vi "Do Something.vi"(8 "error in (no error)":errorcluster, 10 "Bytes to Read":i32, 11 "Inst.Xeryon-Rotator in":refnum<class "Inst.Xeryon-Rotator.lvclass">) -> (0 "error out":errorcluster, 3 "Inst.Xeryon-Rotator out":refnum<class "Inst.Xeryon-Rotator.lvclass">)   [LabVIEW 2019, in "Inst.Xeryon-Rotator.lvclass"]
uses:
  Inst.Xeryon-Rotator.lvclass
  Typedefs/Inst.Xeryon-Rotator.Commands--Enum.ctl
  <userlib>/LevyLab/Instrument Framework/Instrument/Instrument.lvclass
  C:/Program Files (x86)/National Instruments/LabVIEW 2019/user.lib/LevyLab/Instrument Framework/Instrument Types/Cryostat/Instrument.Cryostat.lvclass
  C:/Program Files (x86)/National Instruments/LabVIEW 2019/user.lib/LevyLab/Instrument Framework/Instrument/Instrument.lvclass
  C:/Program Files (x86)/National Instruments/LabVIEW 2019/vi.lib/JKI/JKI SMO/SMO/SMO.lvclass
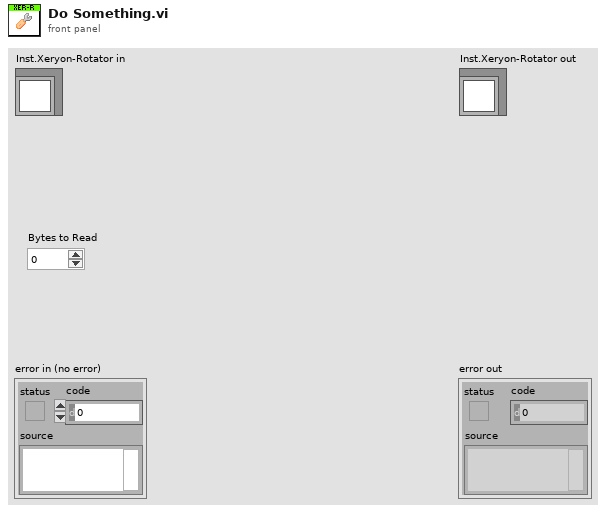
[diagram p1: front panel]
types:
  T1 = typedef "Inst.Xeryon-Rotator.lvclass/Inst.Xeryon-Rotator.Commands--Enum.ctl" = enum16{"setAngle", "getAngle", "setState"}
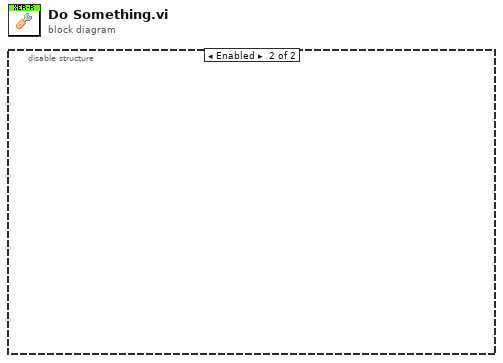
[diagram p0: block diagram]
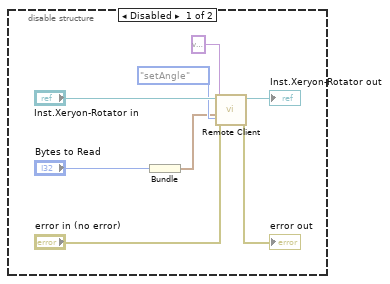
[diagram p2: hidden frame]
diagram:
  n1 = disable-structure shown="Enabled" {
    frame Disabled {
      n2 = Bundle("Bytes to Read"="Bytes to Read") -> (w2:cluster{"Bytes to Read":i32})  [unwired: 1 in]
      n3 = call <userlib>:"Remote Client.vi"("timeout (ms) [500]"=Inst.Xeryon-Rotator.Commands--Enum."setAngle" ("Commands"), "error in (no error)"="error in (no error)", "Data in"=w2, "Command in"=variant ("Data Out type"), "Instrument in"="Inst.Xeryon-Rotator in") -> ("error out"=→"error out":errorcluster, "Instrument out"=→"Inst.Xeryon-Rotator out":refnum<class "Inst.Xeryon-Rotator.lvclass">)  [unwired: 3 in, 2 out]
    }
    frame Enabled {
    }
  }
